vi "Self Attributes.vi"(11 "Base Sender in":refnum<class "Base Sender.lvclass">) -> (2 "Self Attributes":T1)   [LabVIEW 2021, in "jettl.lvlib" / "Sender.lvlib" / "Base Sender.lvclass"]
uses:
  Base Sender.lvclass
  Actor/Attributes.ctl
  Msg/Msg.lvclass
  Actor/Implemented Msgs.ctl
  Base Sender.lvclass/Base Sender.ctl
  Actor/Actor.lvlib
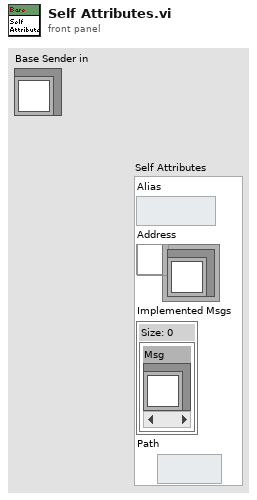
[diagram p1: front panel]
types:
  T1 = typedef "jettl.lvlib/Actor.lvlib/Attributes.ctl" = cluster{"Alias":string, "Address":refnum<user-event>, "Implemented Msgs":T2, "Path":path}
  T2 = typedef "jettl.lvlib/Actor.lvlib/Implemented Msgs.ctl" = set{refnum<class "Msg.lvclass">}
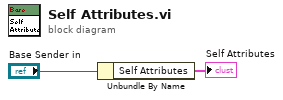
[diagram p0: block diagram]
diagram:
  n1 = Unbundle By Name("Base Sender in") -> ("Self Attributes"=→"Self Attributes":T1)
